vi "build_msg.vi"(9 "data":u8[](array[numeric]), 10 "ID":u16, 11 "Address":u16) -> (3 "msg":u8[](array[numeric]))   [LabVIEW 2014]
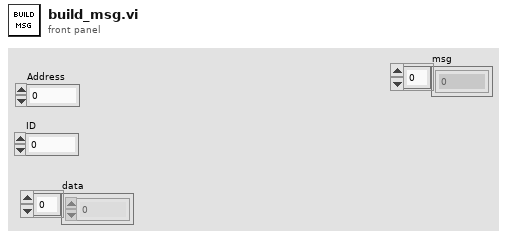
[diagram p1: front panel]
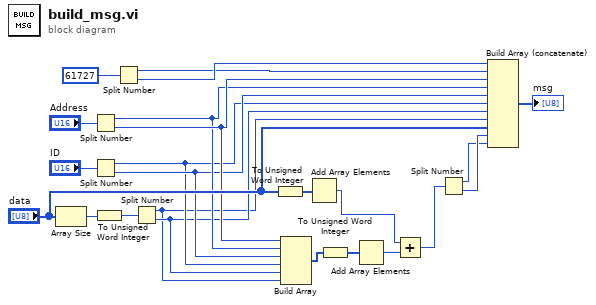
[diagram p0: block diagram]
diagram:
  n1 = Array Size(array="data") -> (size(s)=w18:i32)
  n2 = Split Number(x="Address") -> (hi(x)=w10:u8, lo(x)=w11:u8)
  n3 = Split Number(x="ID") -> (hi(x)=w8:u8, lo(x)=w9:u8)
  n4 = To Unsigned Word Integer(number=w18) -> (unsigned 16bit integer=w17:u16)
  n5 = Split Number(x=u16 61727) -> (hi(x)=w20:u8, lo(x)=w21:u8)
  n6 = Split Number(x=w17) -> (hi(x)=w1:u8, lo(x)=w2:u8)
  n7 = To Unsigned Word Integer(number="data") -> (unsigned 16bit integer=w15:u16[])
  n8 = Build Array(w11, w10, w9, w8, w2, w1) -> (w7:u8[])
  n9 = Add Array Elements(numeric array=w15) -> (sum=w4:u16)
  n10 = To Unsigned Word Integer(number=w7) -> (unsigned 16bit integer=w6:u16[])
  n11 = Add Array Elements(numeric array=w6) -> (sum=w5:u16)
  n12 = Add(x=w4, y=w5) -> (x+y=w3:u16)
  n13 = Split Number(x=w3) -> (hi(x)=w13:u8, lo(x)=w14:u8)
  n14 = Build Array (concatenate)(w21, w20, w11, w10, w9, w8, w2, w1, "data", w14, w13) -> (→"msg":u8[])
